vi "SDCP SMF Rx Logger - FGV (version 1.1).vi"(0 "Command":T2(ring), 1 "error in (no error)":errorcluster) -> (2 "Logged data":T1[](array[typedef]), 3 "Instantaeneous data":T1[](array[typedef]), 4 "error out":errorcluster)   [LabVIEW 2020]
uses:
  Typedefs/SDCP SMF logger - SMF with timestamp.ctl
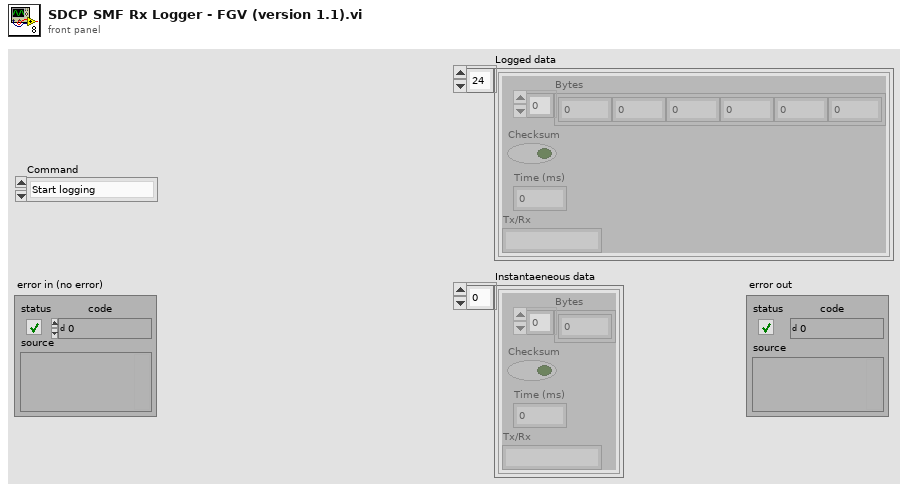
[diagram p1: front panel]
types:
  T1 = typedef "SDCP SMF logger - SMF with timestamp.ctl" = cluster{"Bytes":u8[], "Checksum":bool, "Time (ms)":u32, "Tx/Rx":string}
  T2 = enum16{"Start logging", "Get log data", "Stop logging"}
  T3 = enum16{"Initialize", "Read", "Write", "Deinitialize"}
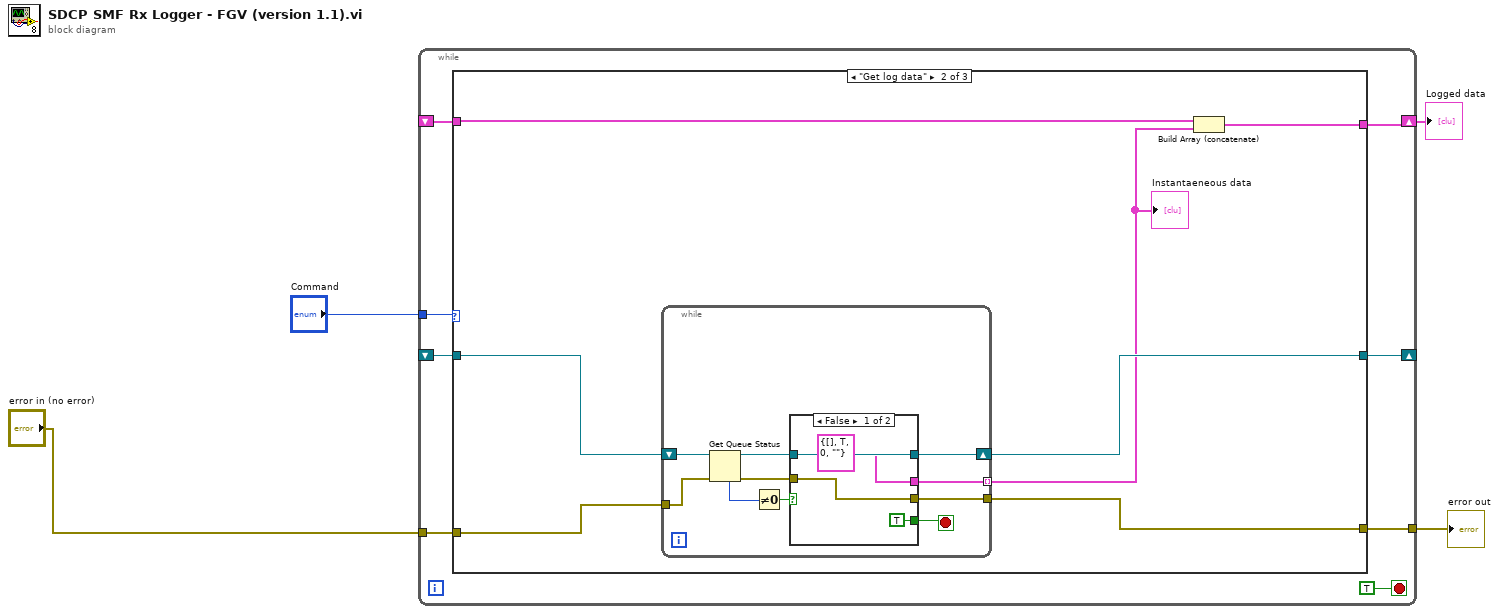
[diagram p0: block diagram]
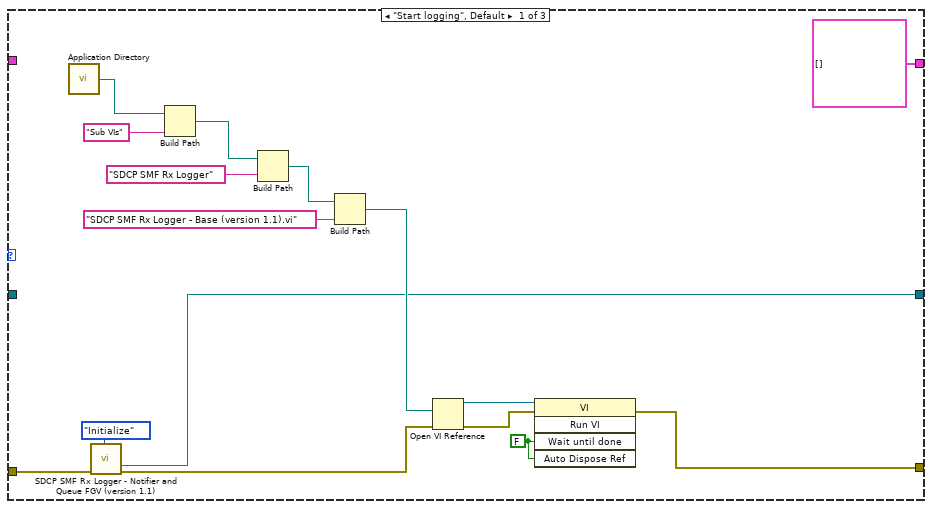
[diagram p2: hidden frame]
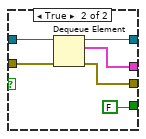
[diagram p3: hidden frame]
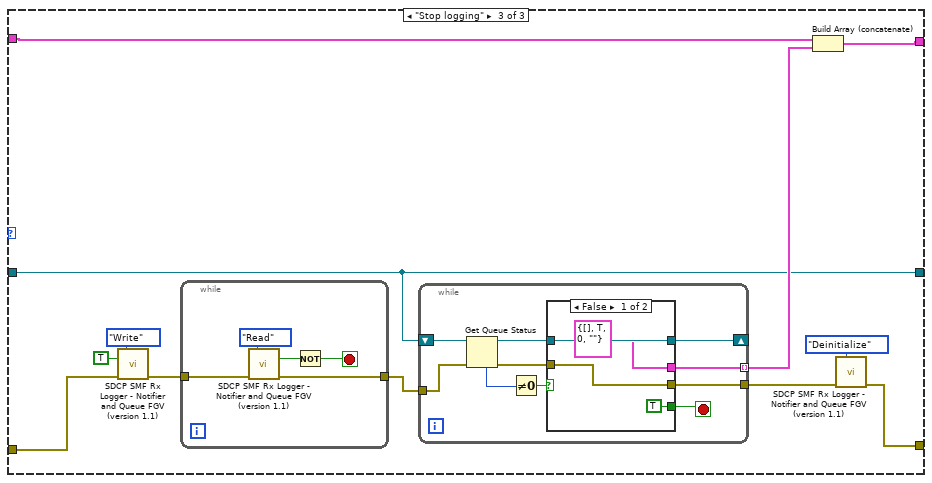
[diagram p4: hidden frame]
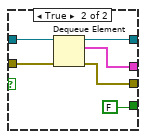
[diagram p5: hidden frame]
diagram:
  n1 = while {
    tunnel: "error in (no error)" -> [w11]
    tunnel: "Command" -> [w10]
    tunnel: [w9] -> w3
    shift-right: [w8] -> _
    shift-left: _ -> [w7]
    shift-right: [w5] -> w2
    shift-left: _ -> [w6]
    stop <- TRUE stop-if-true
    n2 = case shown="\"Get log data\"" w10 {
      tunnel: w11 -> [w28 w35 w67]
      tunnel: [w15 w32 w58] -> w9
      tunnel: [w14 w33 w56] -> w8
      tunnel: w7 -> [_ w34 w56]
      tunnel: w6 -> [_ w31 w62]
      tunnel: [T1[] [] w29 w61] -> w5
      frame "Start logging", Default {
        w16 = FALSE ("Wait Until Done")
        n3 = call <vilib>:"Application Directory.vi"() -> ("Application Directory"=w26:path)
        n4 = call "SDCP SMF Rx Logger - Notifier and Queue FGV (version 1.1).vi"("Commands"=T3."Initialize", "error in (no error)"=w28) -> ("Queue out"=w14:refnum<queue>, "error out"=w19:errorcluster)  [unwired: 9 in, 3 out]
        n5 = Build Path(base path=w26, name or relative path="Sub VIs") -> (appended path=w24:path)
        n6 = Build Path(base path=w24, name or relative path="SDCP SMF Rx Logger") -> (appended path=w22:path)
        n7 = Build Path(base path=w22, name or relative path="SDCP SMF Rx Logger - Base (version 1.1).vi") -> (appended path=w20:path)
        n8 = Open VI Reference(vi path=w20, error in (no error)=w19) -> (vi reference=w18:refnum<vi>, error out=w17:errorcluster)  [unwired: 4 in]
        n9 = invoke class="VI" method="Run VI"(reference=w18, error in=w17, "Wait until done"=w16, "Auto Dispose Ref"=w16) -> (error out=w15:errorcluster)  [unwired: 1 in, 4 out]
      }
      frame "Get log data" {
        n10 = while {
          tunnel: w35 -> [w44]
          shift-right: [w39] -> w33
          shift-left: w34 -> [w45]
          tunnel: [w38] -> w30 mode=indexing
          tunnel: [w36] -> w32
          stop <- w37 stop-if-true
          n11 = Get Queue Status(queue=w45, error in (no error)=w44) -> (queue out=w40:refnum<queue>, error out=w41:errorcluster, # elements in queue=w43:i32)  [unwired: 1 in, 5 out]
          n12 = Not Equal To 0?(x=w43) -> (x != 0?=w42:bool)
          n13 = case shown="False" w42 {
            tunnel: w41 -> [w46 w55]
            tunnel: w40 -> [w49 w54]
            tunnel: [w49 w53] -> w39
            tunnel: [T1 {"Bytes"=[], "Checksum"=TRUE, "Time (ms)"=0, "Tx/Rx"=""} ("SMF with timestamp") w52] -> w38
            tunnel: [TRUE FALSE] -> w37
            tunnel: [w46 w50] -> w36
            frame False {
            }
            frame True {
              n14 = Dequeue Element(queue=w54, error in (no error)=w55) -> (queue out=w53:refnum<queue>, element=w52:T1, error out=w50:errorcluster)  [unwired: 1 in, 1 out]
            }
          }
        }
        "Instantaeneous data" <- w30
        n15 = Build Array (concatenate)(w31, w30) -> (w29:T1[])
      }
      frame "Stop logging" {
        n16 = call "SDCP SMF Rx Logger - Notifier and Queue FGV (version 1.1).vi"("Commands"=T3."Write", "Notification value in"=TRUE, "error in (no error)"=w67) -> ("error out"=w65:errorcluster)  [unwired: 8 in, 4 out]
        n17 = while {
          tunnel: w65 -> [w91]
          tunnel: [w88] -> w64
          stop <- w89 stop-if-true
          n18 = call "SDCP SMF Rx Logger - Notifier and Queue FGV (version 1.1).vi"("Commands"=T3."Read", "error in (no error)"=w91) -> ("Notifier value output"=w90:bool, "error out"=w88:errorcluster)  [unwired: 9 in, 3 out]
          n19 = Not(x=w90) -> (.not. x?=w89:bool)
        }
        n20 = while {
          tunnel: w64 -> [w76]
          shift-right: [w71] -> _
          shift-left: w56 -> [w77]
          tunnel: [w70] -> w63 mode=indexing
          tunnel: [w68] -> w60
          stop <- w69 stop-if-true
          n21 = Get Queue Status(queue=w77, error in (no error)=w76) -> (queue out=w72:refnum<queue>, error out=w73:errorcluster, # elements in queue=w75:i32)  [unwired: 1 in, 5 out]
          n22 = Not Equal To 0?(x=w75) -> (x != 0?=w74:bool)
          n23 = case shown="False" w74 {
            tunnel: w73 -> [w78 w87]
            tunnel: w72 -> [w81 w86]
            tunnel: [w81 w85] -> w71
            tunnel: [T1 {"Bytes"=[], "Checksum"=TRUE, "Time (ms)"=0, "Tx/Rx"=""} ("SMF with timestamp") w84] -> w70
            tunnel: [TRUE FALSE] -> w69
            tunnel: [w78 w82] -> w68
            frame False {
            }
            frame True {
              n24 = Dequeue Element(queue=w86, error in (no error)=w87) -> (queue out=w85:refnum<queue>, element=w84:T1, error out=w82:errorcluster)  [unwired: 1 in, 1 out]
            }
          }
        }
        n25 = Build Array (concatenate)(w62, w63) -> (w61:T1[])
        n26 = call "SDCP SMF Rx Logger - Notifier and Queue FGV (version 1.1).vi"("Commands"=T3."Deinitialize", "error in (no error)"=w60) -> ("error out"=w58:errorcluster)  [unwired: 9 in, 4 out]
      }
    }
  }
  "error out" <- w3
  "Logged data" <- w2
